vi "Enable Arbitrary Waveform.vi"(8 "error in (no error)":errorcluster, 9 "Packets to Generate":i32, 10 "BLE Waveform Path":path, 11 "IVI Refnum in":refnum<k15>) -> (0 "error out":errorcluster, 2 "waveform name":string, 3 "IVI Refnum out":refnum<k15>)   [LabVIEW 2026, in "Nordic nRF52 DK DTM Test.lvlib"]
uses:
  Nordic nRF52 DK DTM Test.lvlib
  <instrlib>/niRFSGPlayback/niRFSGPlayback Read and Download Waveform From File (1 Wfm, 1 RFSG, TDMS).vi
  <instrlib>/niRFSGPlayback/niRFSGPlayback Set Script to Generate (1 RFSG).vi
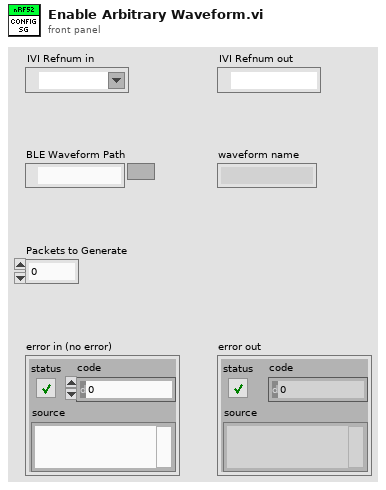
[diagram p1: front panel]
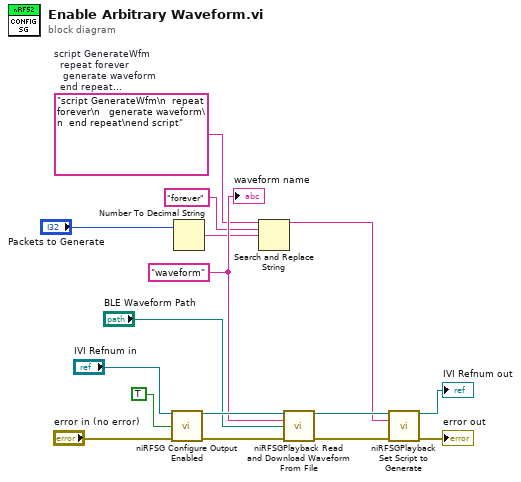
[diagram p0: block diagram]
diagram:
  w8 = "waveform" ("waveform name")
  w1 = "script GenerateWfm\n  repeat forever\n   generate waveform\n  end repeat\nend script"  # script GenerateWfm   repeat forever    generate waveform   end repeat end script
  n1 = call <instrlib>:"niRFSG Configure Output Enabled.vi"("instrument handle"="IVI Refnum in", "output enabled"=TRUE, "error in"="error in (no error)") -> ("instrument handle out"=w16:refnum<k15>, "error out"=w15:errorcluster)  [unwired: 11 in]
  n2 = Number To Decimal String(number="Packets to Generate") -> (decimal integer string=w3:string)  [unwired: 1 in]
  n3 = Search and Replace String(input string=w1, search string="forever", replace string=w3) -> (result string=w5:string)  [unwired: 5 in, 3 out]
  n4 = call-poly <instrlib>:"niRFSGPlayback Read and Download Waveform From File.vi"("instrument handle in"=w16, "waveform name"=w8, "file path"="BLE Waveform Path", "error in"=w15) -> ("instrument handle out"=w10:refnum<k15>, "error out"=w11:errorcluster)  [unwired: 10 in]
  n5 = call-poly <instrlib>:"niRFSGPlayback Set Script to Generate.vi"("instrument handle in"=w10, "script text"=w5, "error in"=w11) -> ("instrument handle out"=→"IVI Refnum out":refnum<k15>, "error out"=→"error out":errorcluster)  [unwired: 11 in]
  "waveform name" <- w8
